vi "Menu parsing.vi"(11 "ItemPath 3":string) -> (2 "ItemPath":string, 3 "ItemPath 2":string)   [LabVIEW 2020]
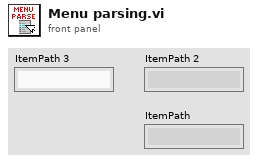
[diagram p1: front panel]
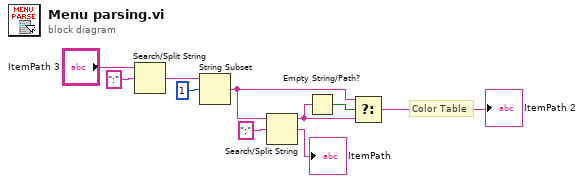
[diagram p0: block diagram]
diagram:
  # "Color Table"
  n1 = Search/Split String(string="ItemPath 3", search string/char (-)=":") -> (match + rest of string=w3:string)  [unwired: 1 in, 2 out]
  n2 = String Subset(string=w3, offset (0)=1) -> (substring=w8:string)  [unwired: 1 in]
  n3 = Search/Split String(string=w8, search string/char (-)=":") -> (substring before match=w7:string, match + rest of string=→"ItemPath":string)  [unwired: 1 in, 1 out]
  n4 = Empty String/Path?(string/path=w7) -> (empty?=w6:bool)
  n5 = Select(t=w8, s=w6, f=w7) -> (s? t:f=→"ItemPath 2":string)
